vi "IR align single.vi"(8 "error in (no error)":errorcluster) -> (0 "error out":errorcluster)   [LabVIEW 2019]
uses:
  distance measure/IR/IR out.ctl
  <vilib>/Platform/TimedLoop/XDataNode/timing_clust.ctl
  <vilib>/Platform/TimedLoop/XDataNode/nitl_modes.ctl
  <vilib>/Platform/TimedLoop/XDataNode/wakeup.ctl
  alignment benchmark.ctl
  <vilib>/platform/TimedLoop/XDataNode/XDataNode.xnode
  <vilib>/Platform/TimedLoop/XDataNode/XDNodeRunTimeDep.lvlib
panel:
  in  "stop":bool
  out "distance out":T1
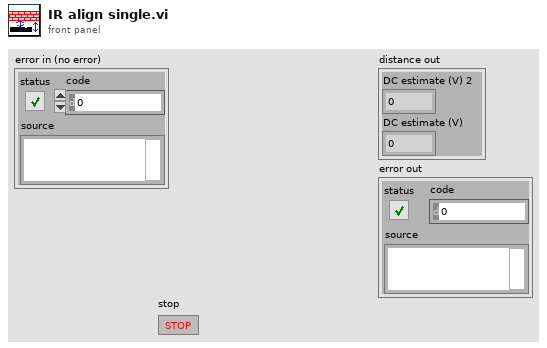
[diagram p1: front panel]
types:
  T1 = typedef "IR out.ctl" = cluster{"DC estimate (V) 2":dbl, "DC estimate (V)":dbl}
  T2 = typedef "alignment benchmark.ctl" = cluster{"DC estimate (V)2":dbl, "DC estimate (V)1":dbl}
  T3 = typedef "XDNodeRunTimeDep.lvlib/timing_clust.ctl" = cluster{"Expected End [f-1]":u64, "Actual End [f-1]":u64, "Finished Late? [f-1]":bool, "Expected End [i-1]":u64, "Actual End [i-1]":u64, "Finished Late? [i-1]":bool, "Expected Start [i]":u64, "Actual Start [i]":u64, "Expected Start [f]":u64, "Actual Start [f]":u64, "Source Name":string, "Structure Name":string, "Period":i64, "Deadline":i64, "Offset":i64, "Start":i64, "Priority":i32, "Timeout":i32, "Mode":T4, "Wakeup Reason":T5, "Error":errorcluster, "Source Type":string, "Secondary Source Type":string, "Global End Time":u64, "Global Start Time":u64, "Frame Duration":u64, "Iteration Duration":u64, "Assigned CPU":i32, "I/O Scan Engine Mode":u32}
  T4 = typedef "XDNodeRunTimeDep.lvlib/nitl_modes.ctl" = enum32{"No Change", "Process missed periods, maintain original phase", "Discard missed periods, maintain original phase", "Process missed periods, ignore original phase", "Discard missed periods, ignore original phase"}
  T5 = typedef "XDNodeRunTimeDep.lvlib/wakeup.ctl" = enum32{"Normal", "Aborted", "Asynchronous wakeup", "Timing source error", "Timed loop error", "Timeout"}
  T6 = typedef "AI.lvlib/AI Reference.ctl" = cluster{"myRIO Reference":T7, "AI Channels List":T11, "AI Scaling Constants List":T13}
  T7 = typedef "myRIO Generic Hardware Reference.ctl" = cluster{"myRIO Model":T8, "myRIO Hardware Reference":T9}
  T8 = typedef "Hardware Version Enum.ctl" = enum16{"Unknown", "myRIO-1900", "myRIO-1950", "roboRIO", "NI ELVIS RIO CM", "ELVIS III"}
  T9 = typedef "myRIO v1.0 Reference.ctl" = cluster{"Generic FPGA Reference":T10, "Allow multiple opens":bool}
  T10 = typedef "Generic FPGA Reference.ctl" = refnum<k20>
  T11 = typedef "AI Channels List.ctl" = T12[]
  T12 = typedef "AI Channels Enum.ctl" = enum16{"Not Connected", "AudioIn/Left", "AudioIn/Right", "C/AI0", "C/AI1", "A/AI0", "A/AI1", "A/AI2", "A/AI3", "A/AI4", "A/AI5", "A/AI6", "A/AI7", "B/AI0", "B/AI1", "B/AI2", "B/AI3", "B/AI4", "B/AI5", "B/AI6", "B/AI7", "AI/AI0", "AI/AI1", "AI/AI2", "AI/AI3", "A/AI0 (DIFF)", "A/AI1 (DIFF)", "A/AI2 (DIFF)", "A/AI3 (DIFF)", "B/AI0 (DIFF)", "B/AI1 (DIFF)", "B/AI2 (DIFF)", "B/AI3 (DIFF)"}
  T13 = typedef "Analog Scaling Constants List.ctl" = T14[]
  T14 = typedef "Analog Scaling Constants.ctl" = cluster{"LSB Weight (Volts)":dbl, "Offset (Volts)":dbl, "Signed?":bool}
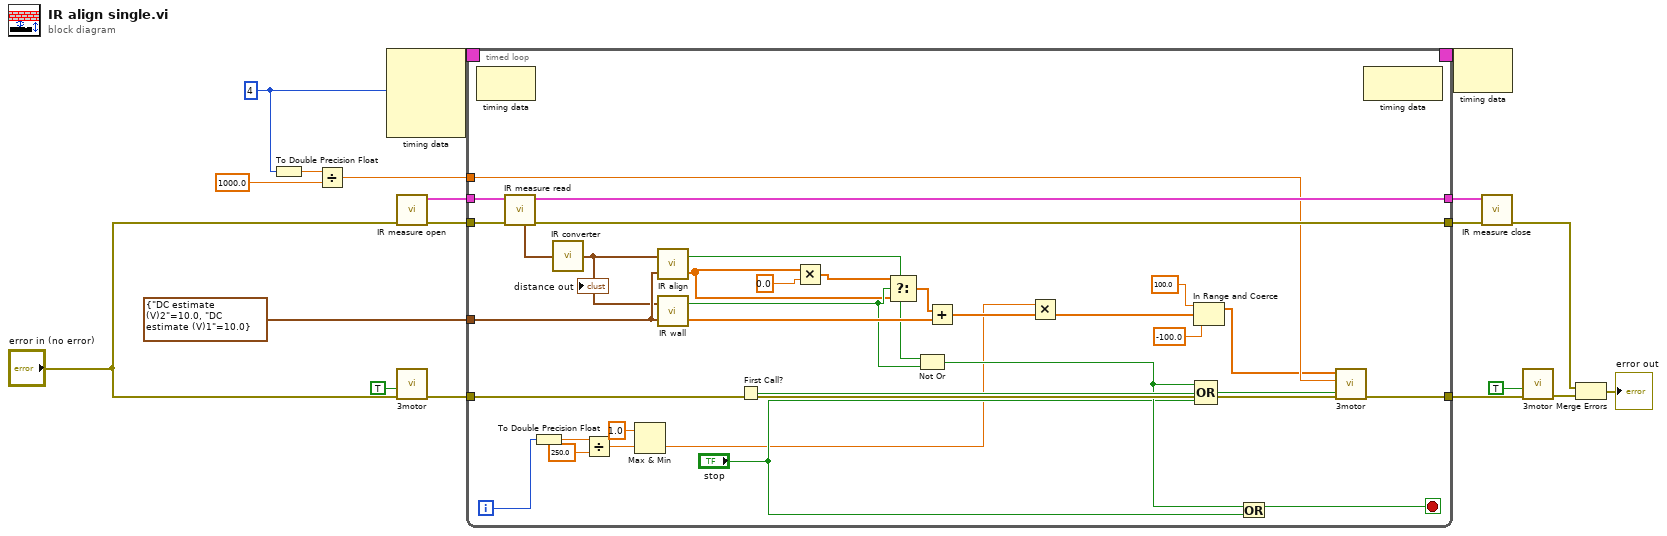
[diagram p0: block diagram]
diagram:
  w10 = i64 4 ("Period")
  n1 = To Double Precision Float(number=w10) -> (double precision float=w9:dbl)
  n2 = Divide(x=w9, y=1000.0) -> (x/y=w7:dbl)
  n3 = node-c288(w10) -> (w17:T3)  [unwired: 3 in]
  n4 = call "IR measure open.vi"("error in (no error)"="error in (no error)") -> ("error out"=w19:errorcluster, "AI Ref Out"=w18:T6)  [unwired: 9 in]
  n5 = call "3motor.vi"("error in (no error)"="error in (no error)", "Reset"=TRUE) -> ("error out"=w11:errorcluster)  [unwired: 9 in]
  n6 = timed-loop {
    timing: w17 -> [_]
    timing-out: [_] -> w16
    tunnel: w19 -> [w52]
    tunnel: w18 -> [w51]
    tunnel: [w50] -> w15
    tunnel: [w49] -> w14
    tunnel: w11 -> [w48]
    tunnel: w7 -> [w47]
    tunnel: [w46] -> w6
    tunnel: T2 {"DC estimate (V)2"=10.0, "DC estimate (V)1"=10.0} -> [w45]
    i -> [w25]
    stop <- w28 stop-if-true
    n7 = node-c288() -> ()  [unwired: 1 in, 1 out]
    n8 = call "IR measure read.vi"("error in (no error)"=w52, "AI Ref In"=w51) -> ("error out"=w50:errorcluster, "AI Ref Out"=w49:T6, "output cluster"=w29:T1)  [unwired: 6 in, 1 out]
    n9 = To Double Precision Float(number=w25) -> (double precision float=w24:dbl)
    n10 = call "IR converter.vi"("IR in"=w29) -> ("distance out"=w30:T1)
    "distance out" <- w30
    n11 = Divide(x=w24, y=250.0) -> (x/y=w22:dbl)
    n12 = Max & Min(x=1.0, y=w22) -> (min(x,y)=w20:dbl)  [unwired: 1 out]
    n13 = call "IR align.vi"("Banchmark in"=w45, "IR in"=w30) -> ("x*y"=w33:dbl[], "x > y?"=w43:bool)
    n14 = call "IR wall.vi"("Banchmark in"=w45, "IR in"=w30) -> ("result"=w44:dbl[], "x > y?"=w34:bool)
    n15 = First Call?() -> (First Call?: T/F=w41:bool)
    n16 = Multiply(x=w33, y=0.0) -> (x*y=w31:dbl[])
    n17 = Select(t=w31, s=w34, f=w33) -> (s? t:f=w35:dbl[])
    n18 = Not Or(1:w34, 2:w43) -> (0:w40:bool)
    n19 = Add(x=w35, y=w44) -> (x+y=w39:dbl[])
    n20 = Multiply(x=w20, y=w39) -> (x*y=w26:dbl[])
    n21 = In Range and Coerce(upper limit=100.0, x=w26, lower limit=-100.0) -> (coerced(x)=w36:dbl[])  [unwired: 1 out]
    n22 = Compound Arithmetic op=OR(w40, w41, "stop") -> (w42:bool)
    n23 = Or(x=w40, y="stop") -> (x .or. y?=w28:bool)
    n24 = call "3motor.vi"("error in (no error)"=w48, "Reset"=w42, "dt(s)"=w47, "Motor speed"=w36) -> ("error out"=w46:errorcluster)  [unwired: 7 in]
    n25 = node-c288() -> ()  [unwired: 1 in, 1 out]
  }
  n26 = node-c288(w16) -> ()  [unwired: 1 out]
  n27 = call "IR measure close.vi"("error in (no error)"=w15, "AI Ref In"=w14) -> ("error out"=w2:errorcluster)  [unwired: 9 in]
  n28 = call "3motor.vi"("error in (no error)"=w6, "Reset"=TRUE) -> ("error out"=w3:errorcluster)  [unwired: 9 in]
  n29 = Merge Errors(w2, w3) -> (→"error out":errorcluster)
